vi "Timetrace_meas_diag_realtime.vi"(6 "LD Signal":tag, 7 "Refresh in (s)":dbl, 8 "error in (no error)":errorcluster, 9 "Reference Signal":tag, 10 "Sensitivity":T1(ring), 11 "Max frequency (Hz)":dbl) -> (0 "error out":errorcluster, 1 "Sampling frequency":dbl, 2 "Number of samples":i16, 3 "Ref_MLD measurement":dbl[][](array[numeric]))   [LabVIEW 2015]
uses:
  <vilib>/DAQmx/read.llb/DAQmx Read (Analog 2D DBL NChan NSamp).vi
  <vilib>/DAQmx/create/channels.llb/DAQmx Create Channel (AI-Voltage-Basic).vi
  <vilib>/DAQmx/configure/timing.llb/DAQmx Timing (Sample Clock).vi
  <vilib>/DAQmx/miscellaneous.llb/DAQmx Fill In Error Info.vi
  <resource>/objmgr/daqmx.rc
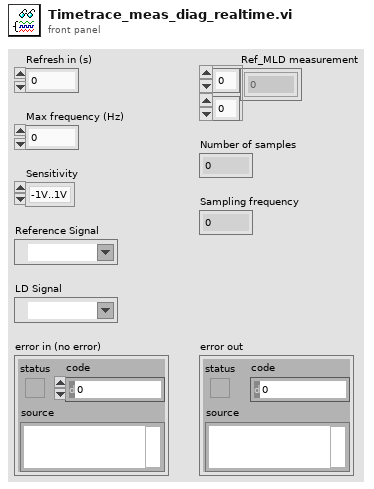
[diagram p1: front panel]
types:
  T1 = enum16{"-1V..1V", "-1.25V..1.25V", "-2V..2V", "-2.5V..2.5V", "-4V..4V", "-5V..5V", "-10V..10V"}
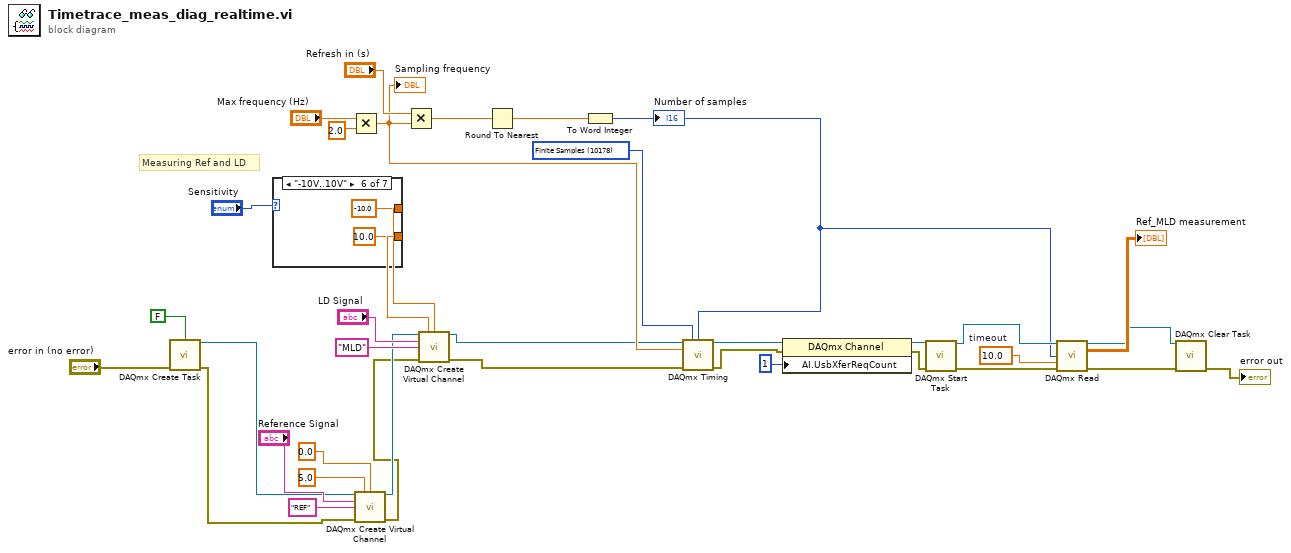
[diagram p0: block diagram]
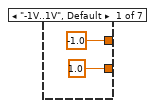
[diagram p2: hidden frame]
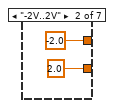
[diagram p3: hidden frame]
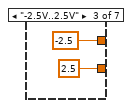
[diagram p4: hidden frame]
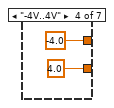
[diagram p5: hidden frame]
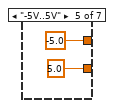
[diagram p6: hidden frame]
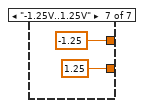
[diagram p7: hidden frame]
diagram:
  w22 = 10.0  # timeout
  w20 = 10178 items=["Finite Samples"=10178, "Continuous Samples"=10123] ("sample mode")
  # "Measuring Ref and LD"
  n1 = call <vilib>:"DAQmx Create Task.vi"("auto cleanup"=FALSE, "error in"="error in (no error)") -> ("task out"=w6:refnum<k21>, "error out"=w5:errorcluster)  [unwired: 12 in]
  n2 = case shown="\"-10V..10V\"" "Sensitivity" {
    tunnel: [-1.0 -2.0 -2.5 -4.0 -5.0 -10.0 -1.25] -> w33
    tunnel: [1.0 2.0 2.5 4.0 5.0 10.0 1.25] -> w34
    frame "-1V..1V", Default {
    }
    frame "-2V..2V" {
    }
    frame "-2.5V..2.5V" {
    }
    frame "-4V..4V" {
    }
    frame "-5V..5V" {
    }
    frame "-10V..10V" {
    }
    frame "-1.25V..1.25V" {
    }
  }
  n3 = Multiply(x="Max frequency (Hz)", y=2.0) -> (x*y=w36:dbl)
  "Sampling frequency" <- w36
  n4 = call-poly <vilib>:"DAQmx Create Virtual Channel.vi"("task in"=w6, "maximum value"=5.0, "minimum value"=0.0, "physical channels"="Reference Signal", "name to assign"="REF", "error in"=w5) -> ("task out"=w4:refnum<k21>, "error out"=w3:errorcluster)  [unwired: 8 in]
  n5 = Multiply(x="Refresh in (s)", y=w36) -> (x*y=w30:dbl)
  n6 = call-poly <vilib>:"DAQmx Create Virtual Channel.vi"("task in"=w4, "maximum value"=w34, "minimum value"=w33, "physical channels"="LD Signal", "name to assign"="MLD", "error in"=w3) -> ("task out"=w2:refnum<k21>, "error out"=w1:errorcluster)  [unwired: 8 in]
  n7 = Round To Nearest(number=w30) -> (nearest integer value=w31:dbl)
  n8 = To Word Integer(number=w31) -> (16bit integer=w14:i16)
  "Number of samples" <- w14
  n9 = call-poly <vilib>:"DAQmx Timing.vi"("task/channels in"=w2, "sample mode"=w20, "samples per channel"=w14, "rate"=w36, "error in"=w1) -> ("task out"=w10:refnum<k21>, "error out"=w8:errorcluster)  [unwired: 9 in]
  n10 = property class="DAQmx Channel"(reference=w10, error in=w8, "AI.UsbXferReqCount"=u32 1) -> (reference out=w9:refnum<k21>, error out=w7:errorcluster)
  n11 = call <vilib>:"DAQmx Start Task.vi"("task/channels in"=w9, "error in"=w7) -> ("task out"=w18:refnum<k21>, "error out"=w17:errorcluster)  [unwired: 12 in]
  n12 = call-poly <vilib>:"DAQmx Read.vi"("task/channels in"=w18, "number of samples per channel"=w14, "timeout"=w22, "error in"=w17) -> ("task out"=w19:refnum<k21>, "data"=→"Ref_MLD measurement":dbl[][], "error out"=w21:errorcluster)  [unwired: 9 in]
  n13 = call <vilib>:"DAQmx Clear Task.vi"("task in"=w19, "error in"=w21) -> ("error out"=→"error out":errorcluster)  [unwired: 13 in]
